vi "Device.Init.vi"(8 "error in (no error)":errorcluster, 11 "XYStage.KIM101 in":refnum<class "XYStage.KIM101.lvclass">) -> (0 "error out":errorcluster, 2 "Result":bool, 3 "XYStage.KIM101 out":refnum<class "XYStage.KIM101.lvclass">)   [LabVIEW 2017, in "XYStage.KIM101.lvclass"]
uses:
  XYStage.KIM101.lvclass
  D:/upwork/Laser Measurement Tool/Laser/project/Subsystems/XYStage/XYStage.lvclass
  Typedefs/Resource--Cluster.ctl
  D:/upwork/Laser Measurement Tool/Laser/project/data/Thorlabs.MotionControl.Controls.dll
  data/Thorlabs.MotionControl.Controls.dll
  D:/upwork/Laser Measurement Tool/Laser/project/data/Thorlabs.MotionControl.KCube.InertialMotorCLI.dll
  data/Thorlabs.MotionControl.KCube.InertialMotorCLI.dll
  XYStage/XYStage.lvclass
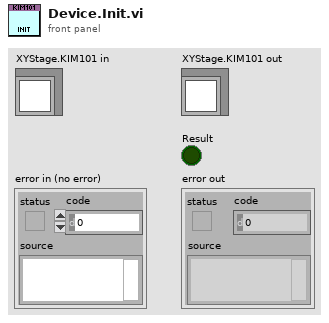
[diagram p1: front panel]
types:
  T1 = typedef "XYStage.KIM101.lvclass/Resource--Cluster.ctl" = cluster{"KCubeInertialMotorControl":refnum<k24>, "Device":refnum<k24>}
  T2 = typedef "XYStage.lvclass/Configuration--Cluster.ctl" = cluster{"Serial Number":string, "X Axis":string, "Y Axis":string, "Real-World Units":string, "Counts per Unit":dbl}
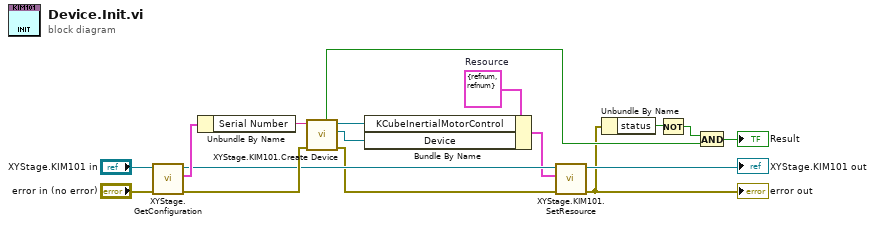
[diagram p0: block diagram]
diagram:
  w12 = T1 {"KCubeInertialMotorControl"=refnum, "Device"=refnum}  # Resource
  n1 = call "XYStage.GetConfiguration.vi"("error in (no error)"="error in (no error)", "XYStage"="XYStage.KIM101 in") -> ("error out"=w13:errorcluster, "Configuration"=w15:T2, "XYStage out"=w9:refnum<class "XYStage.KIM101.lvclass">)  [unwired: 7 in]
  n2 = Unbundle By Name(w15) -> ("Serial Number"=w14:string)
  n3 = call "XYStage.KIM101.Create Device.vi"("error in (no error)"=w13, "SerialNumber"=w14) -> ("error out"=w8:errorcluster, "Device"=w10:refnum<k24>, "KCubeInertialMotorControl"=w11:refnum<k24>, "CreateDevice Result"=w3:bool)  [unwired: 6 in]
  n4 = Bundle By Name(cluster=w12, "KCubeInertialMotorControl"=w11, "Device"=w10) -> (w7:T1)
  n5 = call "XYStage.KIM101.SetResource.vi"("error in (no error)"=w8, "Resource"=w7, "XYStage.KIM101 in"=w9) -> ("error out"=w1:errorcluster, "XYStage.KIM101 out"=→"XYStage.KIM101 out":refnum<class "XYStage.KIM101.lvclass">)  [unwired: 7 in]
  "error out" <- w1
  n6 = Unbundle By Name(w1) -> ("status"=w5:bool)
  n7 = Not(x=w5) -> (.not. x?=w4:bool)
  n8 = And(x=w4, y=w3) -> (x .and. y?=→"Result":bool)
